vi "getDescription.vi"(8 "error in (no error)":errorcluster, 11 "CondimentDecorator in":refnum<class "CondimentDecorator.lvclass">) -> (0 "error out":errorcluster, 2 "description":string, 3 "CondimentDecorator out":refnum<class "CondimentDecorator.lvclass">)   [LabVIEW 2017, in "CondimentDecorator.lvclass"]
uses:
  CondimentDecorator.lvclass
  Beverage Class/Beverage.lvclass
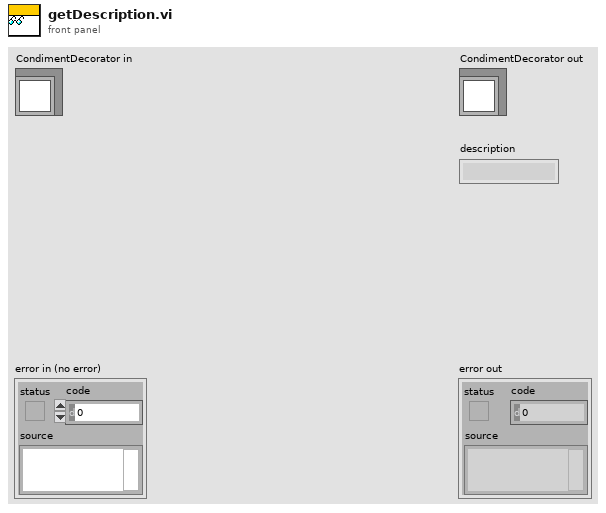
[diagram p1: front panel]
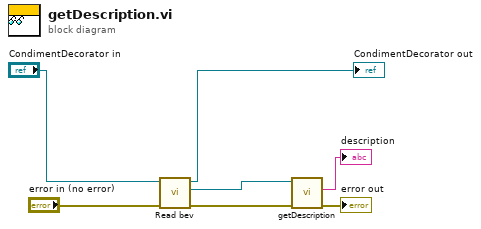
[diagram p0: block diagram]
diagram:
  n1 = call-dynamic "Read bev.vi"("error in (no error)"="error in (no error)", "CondimentDecorator in"="CondimentDecorator in") -> ("error out"=w4:errorcluster, "Beverage.lvclass"=w1:refnum<class "Beverage.lvclass">, "CondimentDecorator out"=→"CondimentDecorator out":refnum<class "CondimentDecorator.lvclass">)  [unwired: 7 in]
  n2 = call-dynamic "getDescription.vi"("error in (no error)"=w4, "Beverage in"=w1) -> ("error out"=→"error out":errorcluster, "description"=→"description":string)  [unwired: 7 in, 1 out]
